vi "自动缩进.vi"(8 "错误输入":errorcluster caption="错误输入（无错误）", 9 "扫描代码":i16, 11 "引用":refnum<k24>) -> (0 "错误输出":errorcluster, 3 "引用输出":refnum<k24>)   [LabVIEW 2018]
uses:
  ScintillaNET.dll
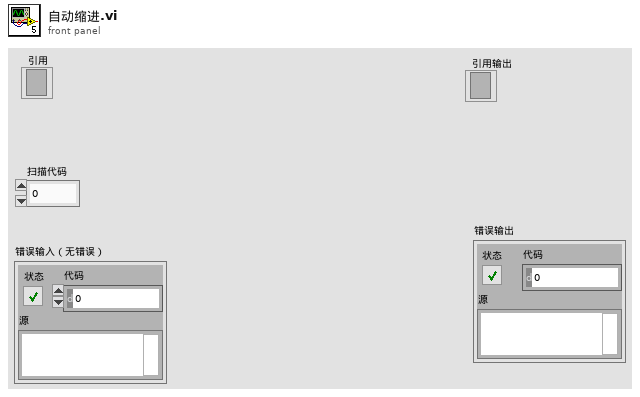
[diagram p1: front panel]
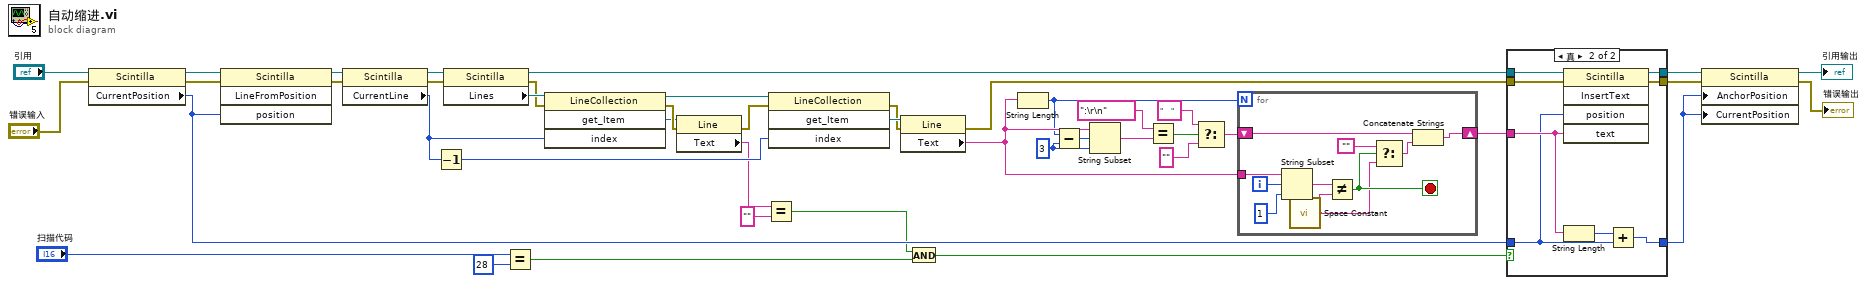
[diagram p0: block diagram]
diagram:
  w14 = 3 ("长度（剩余）")
  n1 = property class="Scintilla"(reference="引用", error in="错误输入") -> (reference out=w42:refnum<k24>, error out=w30:errorcluster, "CurrentPosition"=w41:i32)
  n2 = invoke on="调用节点" class="Scintilla" method="LineFromPosition"(reference=w42, error in=w30, "position"=w41) -> (reference out=w44:refnum<k24>, error out=w29:errorcluster)  [unwired: 1 in, 2 out]
  n3 = property on="属性节点" class="Scintilla"(reference=w44, error in=w29) -> (reference out=w13:refnum<k24>, error out=w28:errorcluster, "CurrentLine"=w1:i32)
  n4 = Decrement(x=w1) -> (x-1=w38:i32)
  n5 = property class="Scintilla"(reference=w13, error in=w28) -> (reference out=w39:refnum<k24>, error out=w8:errorcluster, "Lines"=w10:refnum<k24>)
  n6 = Equal?(x="扫描代码", y=i16 28) -> (x = y?=w3:bool)
  n7 = invoke class="LineCollection" method="get_Item"(reference=w10, error in=w8, "index"=w1) -> (reference out=w9:refnum<k24>, error out=w12:errorcluster, "get_Item"=w11:refnum<k24>)  [unwired: 1 in, 1 out]
  n8 = property class="Line"(reference=w11, error in=w12) -> (error out=w7:errorcluster, "Text"=w6:string)  [unwired: 1 out]
  n9 = Equal?(x=w6, y="") -> (x = y?=w4:bool)
  n10 = invoke class="LineCollection" method="get_Item"(reference=w9, error in=w7, "index"=w38) -> (error out=w27:errorcluster, "get_Item"=w40:refnum<k24>)  [unwired: 1 in, 2 out]
  n11 = property class="Line"(reference=w40, error in=w27) -> (error out=w26:errorcluster, "Text"=w23:string)  [unwired: 1 out]
  n12 = And(x=w4, y=w3) -> (x .and. y?=w2:bool)
  n13 = String Length(string=w23) -> (length=w16:i32)
  n14 = Subtract(x=w16, y=w14) -> (x-y=w15:i32)
  n15 = String Subset(string=w23, offset (0)=w15, length (rest)=w14) -> (substring=w22:string)
  n16 = Equal?(x=":\r\n", y=w22) -> (x = y?=w20:bool)
  n17 = Select(t="    ", s=w20, f="") -> (s? t:f=w19:string)
  n18 = for {
    N: w16 -> [_]
    tunnel: w23 -> [w54]
    shift-right: [w51] -> w35
    shift-left: w19 -> [w50]
    i -> [w52]
    stop <- w49 stop-if-true
    n19 = String Subset(string=w54, offset (0)=w52, length (rest)=1 ("长度（剩余）")) -> (substring=w47:string)
    n20 = call <vilib>:"Space Constant.vi"() -> ("String"=w45:string)
    n21 = Not Equal?(x=w47, y=w45) -> (x != y?=w49:bool)
    n22 = Select(t="", s=w49, f=w45) -> (s? t:f=w48:string)
    n23 = Concatenate Strings(w50, w48) -> (w51:string)
  }
  n24 = case shown="真" w2 {
    tunnel: [w57 w65] -> w34
    tunnel: w41 -> [w56 w61]
    tunnel: w39 -> [w57 w64]
    tunnel: w35 -> [_ w63]
    tunnel: [w56 w60] -> w32
    tunnel: w26 -> [w55 w59]
    tunnel: [w55 w58] -> w25
    frame False {
    }
    frame True {
      n25 = invoke on="调用节点" class="Scintilla" method="InsertText"(reference=w64, error in=w59, "position"=w61, "text"=w63) -> (reference out=w65:refnum<k24>, error out=w58:errorcluster)  [unwired: 1 in, 3 out]
      n26 = String Length(string=w63) -> (length=w62:i32)
      n27 = Add(x=w62, y=w61) -> (x+y=w60:i32)
    }
  }
  n28 = property on="属性节点" class="Scintilla"(reference=w34, error in=w25, "AnchorPosition"=w32, "CurrentPosition"=w32) -> (reference out=→"引用输出":refnum<k24>, error out=→"错误输出":errorcluster)
